vi "SeqMgr.Start Sequence.vi"(8 "error in (no error)":errorcluster, 9 "SeqSteps":string[][](array[string]), 10 "Name":string, 11 "SeqMgr in":refnum<class "SeqMgr.lvclass">) -> (0 "error out":errorcluster, 1 "Start Time":timestamp, 2 "Name":string, 3 "SeqMgr out":refnum<class "SeqMgr.lvclass">)   [LabVIEW 2024, in "EQMF.lvlib" / "SeqMgr.lvlib" / "SeqMgr.lvclass"]
uses:
  SeqMgr.lvclass
  SeqMgr.Progress Type.ctl
  SeqMgr.Result Info.ctl
  SeqMgr.Result State Enum.ctl
  Queues/Q.Msg Return Info.ctl
  Queues/Q.Element.ctl
  SeqMgr.Flow Control Tracking.ctl
  SeqMgr.lvclass/SeqMgr.ctl
  SeqMgr.lvlib
  Queues/Queue Utils.lvlib
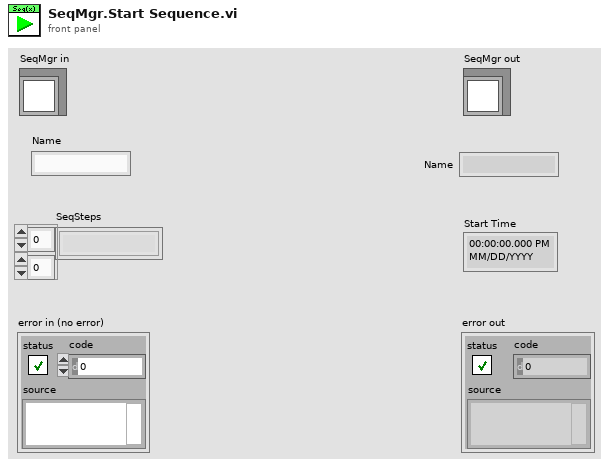
[diagram p1: front panel]
types:
  T1 = typedef "EQMF.lvlib/SeqMgr.lvlib/SeqMgr.Flow Control Tracking.ctl" = cluster{"If Level":i32, "If Index":i32[], "For Level":i32, "For Index":i32[], "While Level":i32, "While Index":i32[], "WRet":bool, "FRet":bool}
  T2 = typedef "EQMF.lvlib/Queue Utils.lvlib/Q.Msg Return Info.ctl" = cluster{"Ret Q":refnum<queue>, "Ret Msg":T3, "SeqNum":i32}
  T3 = typedef "EQMF.lvlib/Queue Utils.lvlib/Q.Element.ctl" = cluster{"Cmd":string, "Sub":string, "Data1":variant, "Data2":variant}
  T4 = typedef "EQMF.lvlib/SeqMgr.lvlib/SeqMgr.Result Info.ctl" = cluster{"State":T5, "Code":i32, "Description":string}
  T5 = typedef "EQMF.lvlib/SeqMgr.lvlib/SeqMgr.Result State Enum.ctl" = enum16{"None", "Passing", "Failing", "PASS", "FAIL", "ABORT", "ERROR"}
  T6 = typedef "EQMF.lvlib/SeqMgr.lvlib/SeqMgr.Progress Type.ctl" = enum16{"Steps", "Time"}
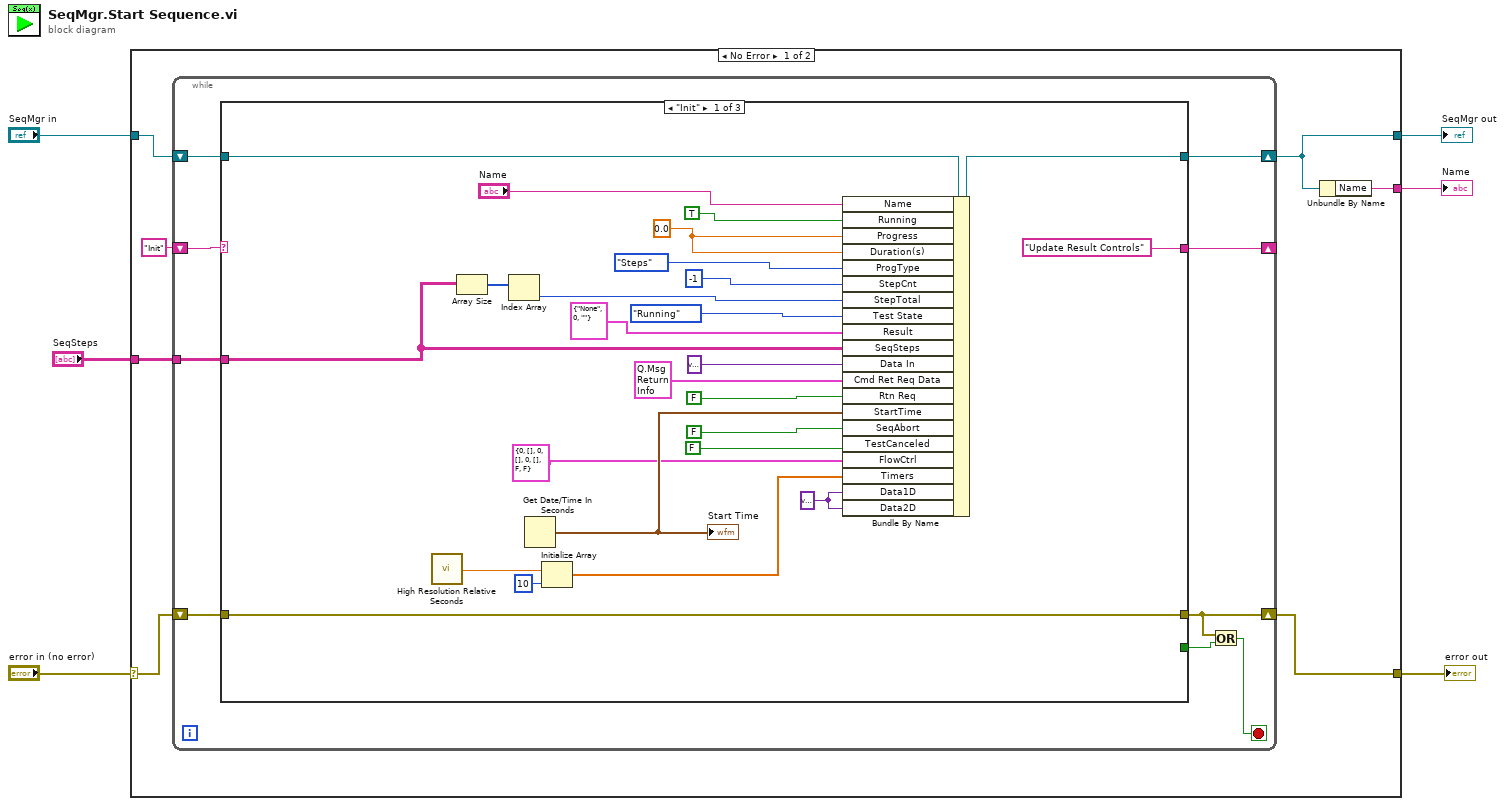
[diagram p0: block diagram]
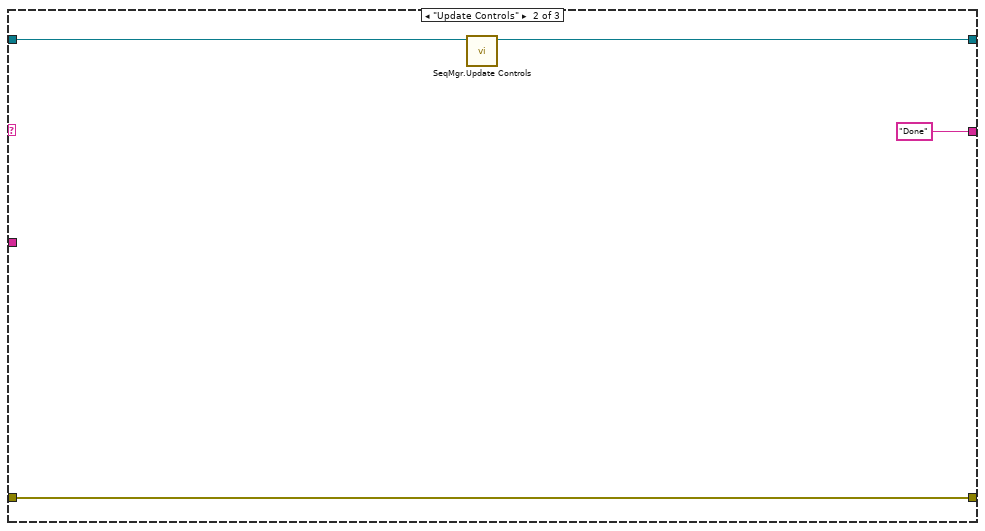
[diagram p2: hidden frame]
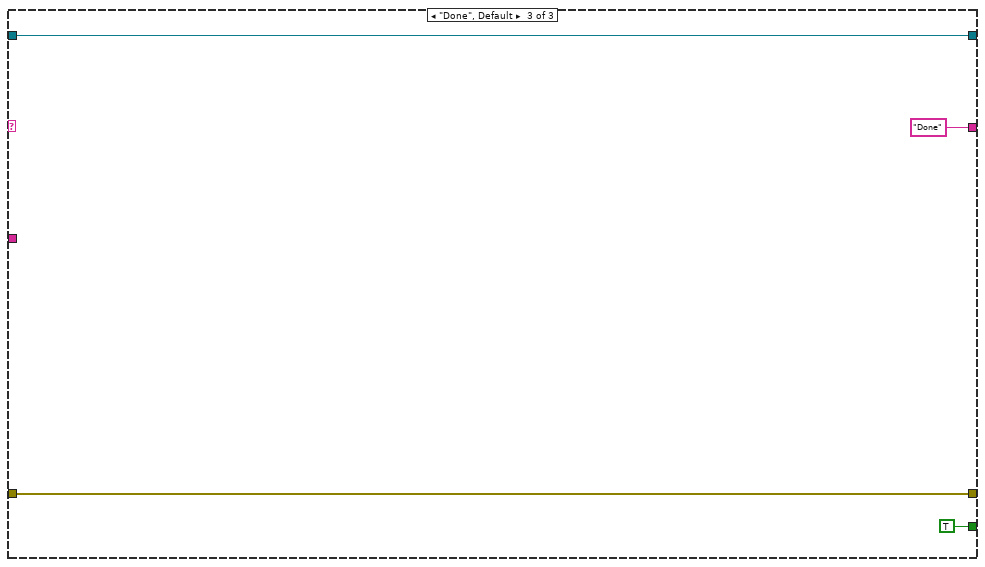
[diagram p3: hidden frame]
diagram:
  n1 = case shown="No Error" "error in (no error)" {
    selector: "error in (no error)" -> [w12 w57]
    tunnel: [w13 w57] -> w5
    tunnel: [w10 w56] -> w3
    tunnel: "SeqMgr in" -> [w11 w56]
    tunnel: "SeqSteps" -> [w7 _]
    tunnel: [w9 _] -> w1
    frame No Error {
      n2 = while {
        shift-right: [w17] -> w10
        shift-left: w11 -> [w22]
        shift-right: [w16] -> _
        shift-left: "Init" -> [w18]
        shift-right: [w20] -> w13
        shift-left: w12 -> [w21]
        tunnel: w7 -> [w14]
        stop <- w19 stop-if-true
        n3 = case shown="\"Init\"" w18 {
          tunnel: w22 -> [w44 w49 w55]
          tunnel: w21 -> [w47 w50 w53]
          tunnel: [w47 w50 w53] -> w20
          tunnel: [w43 w48 w55] -> w17
          tunnel: ["Update Result Controls" "Done" "Done"] -> w16
          tunnel: [_ _ TRUE] -> w15
          tunnel: w14 -> [w35 _ _]
          frame "Init" {
            w23 = variant ("Data1D")
            w40 = 0.0 ("Progress.Progress")
            n4 = call <vilib>:"High Resolution Relative Seconds.vi"() -> ("relative seconds"=w26:dbl)
            n5 = Array Size(array=w35) -> (size(s)=w45:i32[])
            n6 = Index Array(array=w45) -> (element=w39:i32)  [unwired: 1 in]
            n7 = Get Date/Time In Seconds() -> (seconds since 1Jan1904=w30:timestamp)
            "Start Time" <- w30
            n8 = Initialize Array(w26, 10 ("dimension size")) -> (w24:dbl[])
            n9 = Bundle By Name(cluster=w44, "Name"="Name", "Running"=TRUE, "Progress"=w40, "Duration(s)"=w40, "ProgType"=SeqMgr.Progress_Type."Steps" ("Progress.ProgType"), "StepCnt"=-1, "StepTotal"=w39, "Test State"=enum32{"Idle", "Running", "Completed"}."Running" ("Progress.Test State"), "Result"=T4 {"State"=enum."None", "Code"=0, "Description"=""} ("Result Info"), "SeqSteps"=w35, "Data In"=variant, "Cmd Ret Req Data"=T2 {"Ret Q"=refnum, "Ret Msg"={"Cmd"="", "Sub"="", "Data1"=variant, "Data2"=variant}, "SeqNum"=0}, "Rtn Req"=FALSE, "StartTime"=w30, "SeqAbort"=FALSE, "TestCanceled"=FALSE ("SeqAbort"), "FlowCtrl"=T1 {"If Level"=0, "If Index"=[], "For Level"=0, "For Index"=[], "While Level"=0, "While Index"=[], "WRet"=FALSE, "FRet"=FALSE}, "Timers"=w24, "Data1D"=w23, "Data2D"=w23) -> (w43:refnum<class "SeqMgr.lvclass">)
          }
          frame "Update Controls" {
            n10 = call "SeqMgr.Update Controls.vi"("SeqMgr in"=w49) -> ("SeqMgr out"=w48:refnum<class "SeqMgr.lvclass">)  [unwired: 9 in, 1 out]
          }
          frame "Done", Default {
          }
        }
        n11 = Or(x=w20, y=w15) -> (x .or. y?=w19:bool)
      }
      n12 = Unbundle By Name(w10) -> ("Name"=w9:string)
    }
    frame Error {
    }
  }
  "error out" <- w5
  "SeqMgr out" <- w3
  "Name" <- w1
